vi "Initialize Spectrum Analyzer.vi"(8 "Error In":errorcluster, 11 "Audio Analyzer In":refnum<class "Audio Analyzer.lvclass">) -> (0 "Error Out":errorcluster, 3 "Audio Analyzer Out":refnum<class "Audio Analyzer.lvclass">)   [LabVIEW 2021, in "Audio Analyzer.lvclass"]
uses:
  Audio Analyzer.lvclass
  Accessors/Audio Spectrum Notifier/Set Audio Spectrum Notifier.vi
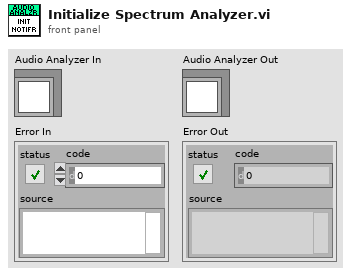
[diagram p1: front panel]
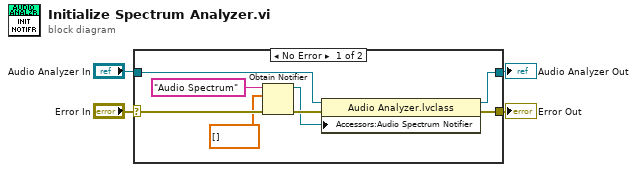
[diagram p0: block diagram]
diagram:
  n1 = case shown="No Error" "Error In" {
    selector: "Error In" -> [w10 w13]
    tunnel: [w5 w13] -> w4
    tunnel: [w6 w14] -> w3
    tunnel: "Audio Analyzer In" -> [w11 w14]
    frame No Error {
      n2 = Obtain Notifier(name (unnamed)="Audio Spectrum", notification data type=dbl[] [], error in (no error)=w10) -> (notifier out=w7:refnum<notifier>, error out=w9:errorcluster)  [unwired: 1 in, 1 out]
      n3 = property class="Audio Analyzer.lvclass"(reference=w11, error in=w9, "Accessors:Audio Spectrum Notifier"=w7) -> (reference out=w6:refnum<class "Audio Analyzer.lvclass">, error out=w5:errorcluster)
    }
    frame Error {
    }
  }
  "Audio Analyzer Out" <- w3
  "Error Out" <- w4
